vi "UHR-Fleezers Control (host) - 11.9c.vi"() -> ()   [LabVIEW 2014] (continued)
  # "Thresholds (nm)"
  # "From FX (nm)"
  # "Break?"
  # "Multiple"
  # "Bad fit"
  # "Hysteresis"
  # "Trap Trig. Fl.?"
  # "1"
  # "2"
  # "Fl. Down"
  # "Fl. Up"
  # "Bead sep"
  # "Trap Display:"
  # "APD Display:"
  # "Trap Manipulation"
  # "Data Saving"
  # "DAQ"
  # "Bead Calibration"
  # "Tether screen"
  # "Bottom Pump (#1)"
  # "Central Sample Channels"
  # "Top Pump (#3)"
  # "Rate param is ul/h\nVolume param is ul"
  # "Chemyx Pump 2"
  # "Units: \n1 = ml/m\n2 = ml/h\n3 = ul/m\n4 = ul/h"
  # "X"
  # "Y"
  # "Oscillate Set 1 freq. (debugging)"
  # "BD 1"
  # "BD 2"
  # "AOD Raster Scan"
  # "Approx. trap separations"
  # "X"
  # "Y"
  # "FPGA\nreading"
  # "DMA\ntransfer"
  # "APD Gates"
  # "APD 2"
  # "APD 1"
  # "X"
  # "2D"
  # "Y"
  # "1D"
  # "Digital Out Control"
  # "Analog Out Control (Feedback Loop)"
  # "Laser Intensity Analog Input"
  # "Total AI Rates (NOT rates/trap)"
  # "(Samples/trap x Trap Sets)"
  # "(Samples/channel x\n8 if averaging (8 channels)\n4 if no averaging)"
  # "Trap 1"
  # "Trap 2"
  # "Flour./Trap 3"
  # "External Video Window"
  # "MCL Position Debugging"
  # "Temporary Control Storage\n(these used to be somewhere else, still want to keep them)"
  # "Y"
  # "X"
  # "Trap Position Difference Limits"
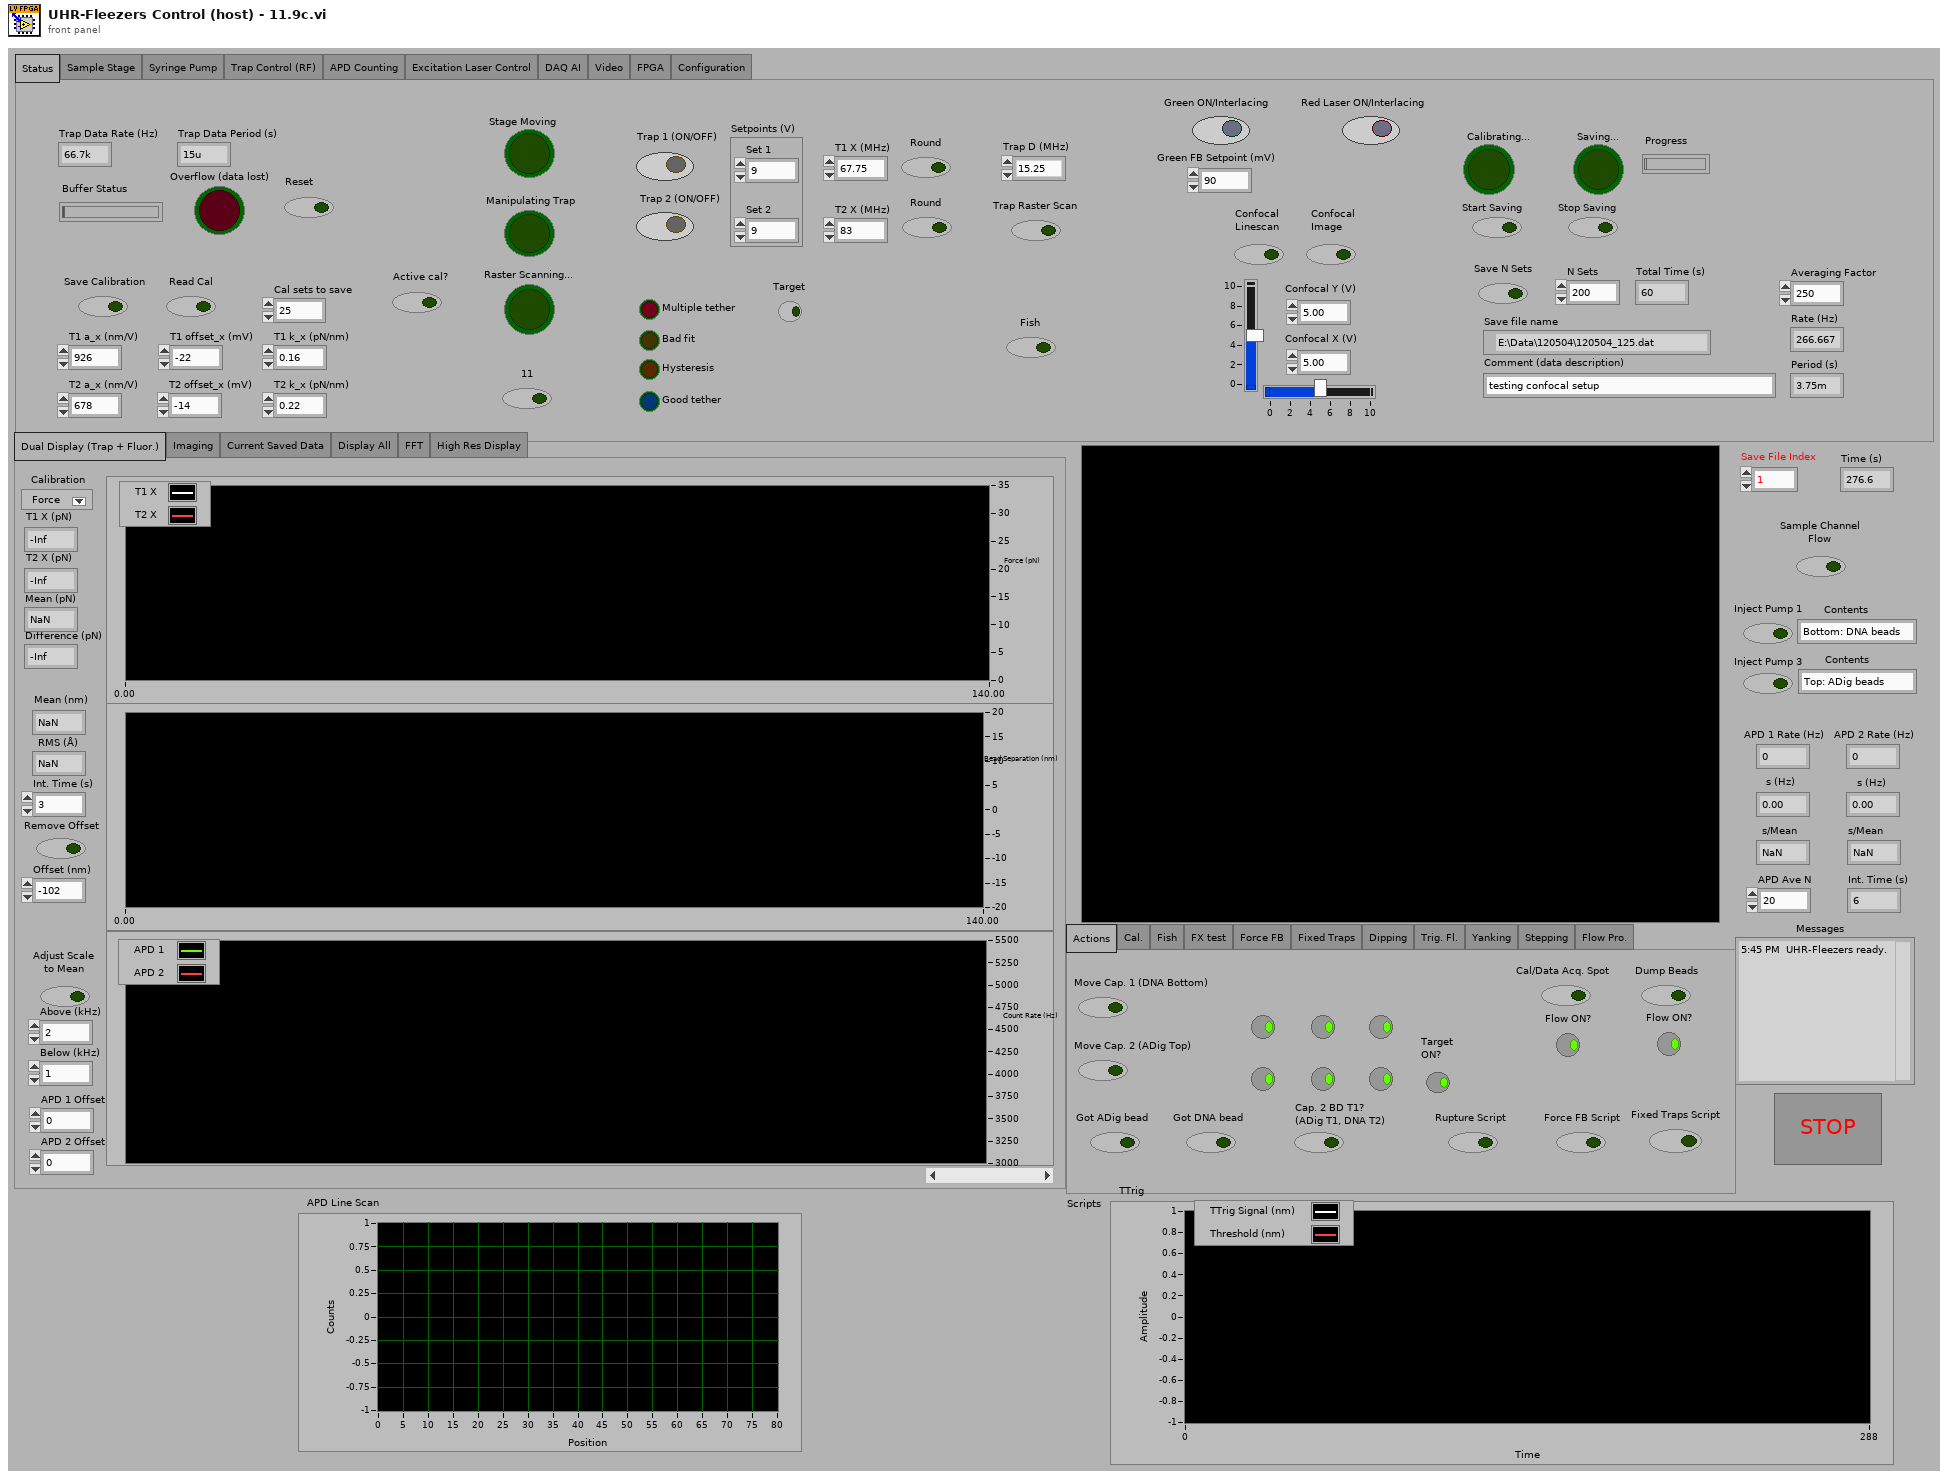
[diagram p1: front panel]
types:
  T1 = enum32{"Actions", "Cal.", "Fish", "FX test", "Force FB", "Fixed Traps", "Dipping", "Trig. Fl.", "Yanking", "Stepping", "Flow Pro."}
  T2 = typedef "IMAQ Image.ctl" = refnum<image>
  T3 = enum32{"Dual Display (Trap + Fluor.)", "Imaging", "Current Saved Data", "Display All", "FFT", "High Res Display"}
  T4 = enum32{"Status", "Sample Stage", "Syringe Pump", "Trap Control (RF)", "APD Counting", "Excitation Laser Control", "DAQ AI", "Video", "FPGA", "Configuration"}
  T5 = cluster{"Pump 1":cluster{"Diameter (mm)":dbl, "Units":dbl, "Volume":dbl, "Rate":dbl}, "Pump 2":cluster{"Diameter (mm)":dbl, "Units":dbl, "Volume":dbl, "Rate":dbl}, "Pump 3":cluster{"Diameter (mm)":dbl, "Units":dbl, "Volume":dbl, "Rate":dbl}}
  T6 = enum32{"IR Laser Interlacing (Direct RF Board Control Method)", "AOD Raster Scan", "Feedback on Trap Intensity", "Feedback on Trap Position"}
  T7 = typedef "LVPoint32TypeDef.ctl" = cluster{"Horizontal":i32, "Vertical":i32}
  T8 = cluster{"Scan Range AOD (nm) 2":dbl, "Step Size AOD (nm) 2":dbl, "Scan Speed AOD (nm/s) 2":dbl, "Number of scans (AOD) 2":u16, "Label":string}[]
  T9 = cluster{"Set 1":cluster{"proportional gain (Kc)":i16, "integral gain (Kc*Ts/Ti)":i16, "derivative gain (Kc*Td/Ts)":i16}, "Set 2":cluster{"proportional gain (Kc)":i16, "integral gain (Kc*Ts/Ti)":i16, "derivative gain (Kc*Td/Ts)":i16}}
  T10 = cluster{"Trap 1":fxp<+/-,16,1>, "Trap 2":fxp<+/-,16,1>}
  T11 = cluster{"proportional gain (Kc)":fxp<+/-,16,8>, "integral gain (Kc*Ts/Ti)":fxp<+/-,16,8>, "derivative gain (Kc*Td/Ts)":fxp<+/-,16,8>}
  T12 = cluster{"output high":fxp<+/-,64,32>, "output low":fxp<+/-,64,32>}
  T13 = cluster{"Set 1":fxp<+/-,16,1>, "Set 2":fxp<+/-,16,1>}
  T14 = enum32{"Main Controls", "Green laser (532 nm)", "Red laser (633 nm)"}
  T15 = cluster{"proportional gain (Kc)":i16, "integral gain (Kc*Ts/Ti)":i16, "derivative gain (Kc*Td/Ts)":i16}
  T16 = cluster{"Set 1":bool, "Set 2":bool, "Set 3":bool}
  T17 = typedef "LVMinMaxIncTypeDef.ctl" = cluster{"Minimum":dbl, "Maximum":dbl, "Increment":dbl}
  T18 = typedef "Image Type" = u32
  T19 = typedef "nirio_resource_hc.ctl" = tag
  T20 = typedef "openfpgaref.8.6.ctl" = refnum<k20>
  T21 = cluster{"New Image":T2, "New Image":T2, "New Image":T2, "New Image":T2}
  T22 = typedef "XDNodeRunTimeDep.lvlib/timing_clust.ctl" = cluster{"Expected End [f-1]":u64, "Actual End [f-1]":u64, "Finished Late? [f-1]":bool, "Expected End [i-1]":u64, "Actual End [i-1]":u64, "Finished Late? [i-1]":bool, "Expected Start [i]":u64, "Actual Start [i]":u64, "Expected Start [f]":u64, "Actual Start [f]":u64, "Source Name":string, "Structure Name":string, "Period":i64, "Deadline":i64, "Offset":i64, "Start":i64, "Priority":i32, "Timeout":i32, "Mode":T23, "Wakeup Reason":T24, "Error":errorcluster, "Source Type":string, "Secondary Source Type":string, "Global End Time":u64, "Global Start Time":u64, "Frame Duration":u64, "Iteration Duration":u64, "Assigned CPU":i32, "I/O Scan Engine Mode":u32}
  T23 = typedef "XDNodeRunTimeDep.lvlib/nitl_modes.ctl" = enum32{"No Change", "Process missed periods, maintain original phase", "Discard missed periods, maintain original phase", "Process missed periods, ignore original phase", "Discard missed periods, ignore original phase"}
  T24 = typedef "XDNodeRunTimeDep.lvlib/wakeup.ctl" = enum32{"Normal", "Aborted", "Asynchronous wakeup", "Timing source error", "Timed loop error", "Timeout"}
  T25 = enum16{"big-endian, network order", "native, host order", "little-endian"}
  T26 = enum16{"open", "replace", "create", "open or create", "replace or create", "replace or create with confirmation"}
  T27 = cluster{"Scan Range AOD (nm) 2":dbl, "Step Size AOD (nm) 2":dbl, "Scan Speed AOD (nm/s) 2":dbl, "Number of scans (AOD) 2":u16, "Label":string}
  T28 = cluster{"[0]":dbl, "[1]":dbl, "[2]":dbl, "[3]":dbl, "[4]":dbl, "[5]":dbl}
  T29 = cluster{"Diameter (mm)":dbl, "Units":dbl, "Volume":dbl, "Rate":dbl}
  T30 = enum16{"Actions", "Cal.", "Fish", "FX test", "Force FB", "Fixed Traps", "Dipping", "Trig. Fl.", "Yanking", "Stepping", "Flow Pro."}
  T31 = cluster{"Left":i32, "Top":i32, "Width":u32, "Height":u32}
  T32 = cluster{cluster{"Left":i32, "Top":i32, "Width":u32, "Height":u32}}[]
  T33 = enum32{"setting", "request", "request control", "info", "statistics", "system settings", "I/O sub system", "HRT control", "camera descriptions", "device specific data", "event sub system settings", "event sub system results", "image memory manager"}
  T34 = typedef "AviRefnum.ctl" = refnum<k1>
  T35 = typedef "imagedata.ctl" = cluster{"image type":i32, "image depth":i32, "image":u8[], "mask":u8[], "colors":u32[], "Rectangle":cluster{"left":i16, "top":i16, "right":i16, "bottom":i16}}
  T36 = enum32{"Normal Display", "Dual Display (APD)", "FFT", "High Res Display"}
  T37 = cluster{"Origin Pixel":cluster{"X":sgl, "Y":sgl}, "Angle Relative to Horizontal (deg)":sgl, "Axis Reference":u32}
  T38 = typedef "Simple Grid Descriptor" = cluster{"X Step":sgl, "Y Step":sgl, "Unit":T39}
  T39 = typedef "Image Unit" = enum32{"Undefined", "Angström", "Micrometer", "Millimeter", "Centimeter", "Meter", "Kilometer", "Microinch", "Inch", "Feet", "Nautical miles", "Standard miles", "Steps"}
  T40 = cluster{"averaging mode":u16, "weighting mode":u16, "number of averages":u32}
  T41 = cluster{"dB On (F)":bool, "unwrap phase (F)":bool, "convert to degree (F)":bool}
  T42 = cluster{string, string, string, string, string, string, string, string}
  T43 = cluster{string, string, string, string, string, string, string, string, string, string, string, string}
  T44 = cluster{string, string, string, string, string, string, string, string, string, string, string, string, string}
  T45 = cluster{string, string, string, string, string, string, string, string, string, string, string, string, string, string}
  T46 = cluster{"BD 1 Frequency 1 (MHz)":dbl, "BD 1 Frequency 2 (MHz)":dbl}
  T47 = cluster{"f0":dbl, "df":dbl, "magnitude":dbl[]}[][]
  T48 = cluster{"Green FB Ch 0":i16, "Green FB Ch 1":i16, "Green FB Ch 2":i16}
  T49 = cluster{"Green FB Ch 0":dbl, "Green FB Ch 1":dbl, "Green FB Ch 2":dbl}
diagram:
  w26 = 0.0 ("Total Volume\nFlowed P1 (uL)")
  w38 = u16 20 items=["1.0"=10, "1.5"=15, "2.0"=20] ("stop bits (10: 1 bit)")
  w41 = u16 20 items=["1.0"=10, "1.5"=15, "2.0"=20] ("stop bits (10: 1 bit)")
  w96 = u16 20 items=["1.0"=10, "1.5"=15, "2.0"=20] ("stop bits (10: 1 bit)")
  w103 = T18 2 items=["Grayscale (U8)", "Grayscale (I16)", "Grayscale (SGL)", "Complex (CSG)", "RGB (U32)", "HSL (U32)", "RGB (U64)", "Grayscale (U16)"] ("Image Type")
  w162 = cluster{"output high":i16, "output low":i16} {"output high"=3000, "output low"=0} ("FB output range 1")
  w233 = 10.0 ("y")
  w232 = 32767.0 ("y")
  w248 = 6.0  # clock mult.
  w249 = 49152000.0  # TCXO frequ.
  # "Safety limits on RF frequencies and amplitudes (for AOM protection)"
  # "Bottom 1 Harvard"
  # "Top 3 Harvard"
  # "Center Harvard"
  # "Bottom 1 Harvard"
  # "Top 3 Harvard"
  # "Center Harvard"
  n1 = Build Array("DIO count 1 (ticks)", "DIO count 2 (ticks)", "DIO count 3 (ticks)") -> (w149:u32[])
  n2 = local read "AO1"() -> (w227:dbl)
  n3 = local read "AO2"() -> (w226:dbl)
  n4 = local read "Scan Increment (MHz)"() -> (w244:dbl)
  n5 = local read "Continuous MCL Scanning"() -> (w214:bool)
  n6 = local read "Fast Scan Dir"() -> (w213:bool)
  n7 = local read "Number of scans (MCL)"() -> (w215:u64)
  n8 = property on="AI Count (ticks)" class="DigNum (strict)"("Val(Sgnl)"="AI Count (ticks)") -> ()  [unwired: 2 in, 2 out]
  n9 = Multiply(x=w227, y=w232) -> (x*y=w229:dbl)
  n10 = Multiply(x=w226, y=w232) -> (x*y=w231:dbl)
  n11 = Divide(x=w229, y=w233) -> (x/y=w228:dbl)
  n12 = Divide(x=w231, y=w233) -> (x/y=w230:dbl)
  n13 = To Word Integer(number=w228) -> (16bit integer=w225:i16)
  n14 = To Word Integer(number=w230) -> (16bit integer=w224:i16)
  n15 = Not(x=w213) -> (.not. x?=w208:bool)
  n16 = local read "Cycles/step (MCL)"() -> (w216:u64)
  n17 = Multiply(x=w244, y=1000.0) -> (x*y=w251:dbl)
  n18 = local read "Scan steps (MCL)"() -> (w217:u64)
  n19 = local write "Trap Pos FIFO Timeout"(u16 0 ("Trap Pos FIFO Timeout")) -> ()
  n20 = local read "Desired Scan Incr (V)"() -> (w219:dbl)
  n21 = Scale By Power Of 2(n=48, x=w251) -> (x*2^n=w252:dbl)
  n22 = Multiply(x=w249, y=w248) -> (x*y=w247:dbl)
  n23 = Divide(x=w252, y=w247) -> (x/y=w246:dbl)
  n24 = local read "Setpoints (V)"() -> (w263:cluster{"Set 1":dbl, "Set 2":dbl})
  n25 = To Quad Integer(1:w246) -> (0:w243:i64)
  n26 = Divide(x=40000000.0, y="AI Count (ticks)") -> (x/y=w204:dbl)
  n27 = Multiply(x=w219, y=32767.0) -> (x*y=w221:dbl)
  n28 = local read "Number Interlace Sets"() -> (w142:u8)
  n29 = Split 1D Array(array=w149, index=w142) -> (first subarray=w151:u32[])  [unwired: 1 out]
  n30 = Add Array Elements(numeric array=w151) -> (sum=w150:u32)
  n31 = local read "# Samples/channel"() -> (w236:u32)
  n32 = local read "Number of F/B Scans (AOD)"() -> (w237:u16)
  n33 = local read "Not-Interlacing Set"() -> (w141:enum32{"Set 1", "Set 2", "Set 3"})
  n34 = To Unsigned Byte Integer(number=w141) -> (unsigned 8bit integer=w147:u8)
  n35 = Index Array(array=w149, index=w147) -> (element=w148:u32)
  n36 = local read "Feedback On/Off"() -> (w266:cluster{"Set 1":bool, "Set 2":bool})
  n37 = local read "PID Gains"() -> (w258:T9)
  n38 = local read "Scan steps (AOD)"() -> (w242:u64)
  n39 = local read "All FB On/Off"() -> (w267:bool)
  n40 = local read "Cycles/step (AOD)"() -> (w241:u64)
  n41 = local write "AI rate (Hz)"(w204) -> ()
  n42 = Divide(x=w221, y=10.0) -> (x/y=w220:dbl)
  n43 = Multiply(x=w242, y=w241) -> (x*y=w240:u64)
  n44 = Multiply(x=3276.7, y=w263) -> (x*y=w262:cluster{"Set 1":dbl, "Set 2":dbl})
  n45 = To Word Integer(number=w220) -> (16bit integer=w218:i16)
  n46 = xnode "Open FPGA VI Reference"("resource name"=T19 "RIO1") -> ("FPGA VI Reference Out"=w24:T20, "error out"=w22:errorcluster)  [unwired: 1 in]
  n47 = Multiply(x=w240, y=u64 2) -> (x*y=w238:u64)
  n48 = local read "Sets to FIFO (Traps)"() -> (w270:T16)
  n49 = Divide(x=w204, y="FPGA Ave.") -> (x/y=w205:dbl)
  n50 = To Word Integer(number=w262) -> (16bit integer=w261:cluster{"Set 1":i16, "Set 2":i16})
  n51 = Unbundle By Name(w258) -> ("Set 1"=w257:T15, "Set 2"=w256:T15)
  n52 = Multiply(x=w238, y=w237) -> (x*y=w235:u64)
  n53 = local write "Ave. Rate (Hz)"(w205) -> ()
  n54 = Divide(x=w235, y=w236) -> (x/y=w234:dbl)
  n55 = Unbundle By Name(w261) -> ("Set 1"=w260:i16, "Set 2"=w259:i16)
  n56 = local read "2D or 1D Scan"() -> (w163:bool)
  n57 = local write "Data points/scans"(w235) -> ()
  n58 = local read "Scan BD"() -> (w253:bool)
  n59 = And(x=w266, y=w267) -> (x .and. y?=w265:cluster{"Set 1":bool, "Set 2":bool})
  n60 = local write "Data points/scan (f/b)"(w238) -> ()
  n61 = Reciprocal(x=w205) -> (1/x=w206:dbl)
  n62 = local read "N Acq Sets (Traps + Fl.)"() -> (w197:i16)
  n63 = local write "N sets should be saved"(w234) -> ()
  n64 = xnode "Invoke Method"("FPGA VI Reference In"=w24, "error in"=w22) -> ("FPGA VI Reference Out"=w161:T20, "error out"=w171:errorcluster)
  n65 = Unbundle By Name(w265) -> ("Set 1"=w269:bool, "Set 2"=w268:bool)
  n66 = local read "Interlace"() -> (w143:bool)
  n67 = Select(t=w150, s=w143, f=w148) -> (s? t:f=w140:u32)
  n68 = local write "Update Count (MCL)"(w140) -> ()
  n69 = local write "Total Counts (ticks)"(w140) -> ()
  n70 = local write "Ave. Period (s)"(w206) -> ()
  n71 = property on="2D or 1D Scan" class="Bool (strict)"("Val(Sgnl)"=w163) -> ()  [unwired: 2 in, 2 out]
  n72 = local read "APD Gate OFF Count"() -> (w65:u16)
  n73 = local read "Interlace OFF count"() -> (w68:u16)
  n74 = local read "Interlace ON count"() -> (w3:u16)
  n75 = local read "APD Gate ON Count"() -> (w61:u16)
  n76 = xnode "Read/Write Control"("FPGA VI Reference In"=w160, "error in"=w171, "ai count"="AI Count (ticks)", "Interlace ON/OFF"=w143, "Number Interlace Cycles"=w142, "AI1 Sets to FIFO"=w270, "FB On/Off Set 1"=w269, "FB On/Off Set 2"=w268, "Interlace Off Parameters"=w141, "FB Setpoint Set 1"=w260, "FB Setpoint Set 2"=w259, "FB Gains Set 1"=w257, "FB Gains Set 2"=w256, "FB output range 1"=w162, "FB output range 2"=w162, "Cycles per step"=w241, "Scan BD"=w253, "Number of scans"=w237, "Scan steps"=w242, "Scan freq.  increment"=w243, "AO1"=w225, "AO2"=w224, "Scan freq.  increment (MCL)"=w218, "Scan steps (MCL)"=w217, "Cycles per step (MCL)"=w216, "Number of scans (MCL)"=w215, "MCL count"=w140, "Cont. Scan (MCL)"=w214, "MCL Scan Axis"=w208, "1D or 2D Scan?"=w163, "N of AI1 Int Acq Sets"=w197, "Freq or Amp switch first"="Freq or Amp switch first", "Freq switch delay"="Freq switch delay", "Amp switch delay"="Amp switch delay", "Swap F1 and F2"="Swap F1 and F2", "APD to FIFO"=FALSE, "DIO count 1 (ticks)"="DIO count 1 (ticks)", "DIO count 2 (ticks)"="DIO count 2 (ticks)", "DIO count 3 (ticks)"="DIO count 3 (ticks)") -> ("FPGA VI Reference Out"=w72:T20, "error out"=w70:errorcluster)  [unwired: 1 in]
  n77 = local read "Duty frequency (ON 1/N cycles)"() -> (w67:u16)
  n78 = local read "APD Integration Time (s)"() -> (w53:dbl)
  n79 = local read "DMA Update Period (s)"() -> (w52:dbl)
  n80 = local read "Red Laser ON/Interlacing"() -> (w6:bool)
  n81 = Add(x=w61, y=w65) -> (x+y=w63:u16)
  n82 = local read "Laser interlacing mode (all lasers)"() -> (w5:enum32{"Laser ON", "Laser OFF", "Interlace"})
  n83 = Add(x=w3, y=w68) -> (x+y=w66:u16)
  n84 = local read "Green ON/Interlacing"() -> (w139:bool)
  n85 = Multiply(x=w63, y=w67) -> (x*y=w64:u16)
  n86 = Multiply(x=w67, y=w66) -> (x*y=w60:u16)
  n87 = Reciprocal(x=w53) -> (1/x=w50:dbl)
  n88 = Multiply(x=w53, y=40000000.0) -> (x*y=w49:dbl)
  n89 = Divide(x=w52, y=w53) -> (x/y=w55:dbl)
  n90 = Multiply(x="Green intensity % (FB OFF)", y=655.35) -> (x*y=w129:dbl)
  n91 = local read "Invert laser interlacing"() -> (w1:bool)
  n92 = case shown="False" w6 {
    tunnel: w5 -> [_ w295]
    tunnel: [enum32{"Laser ON", "Laser OFF", "Interlace"}."Laser OFF" ("Laser interlacing mode (all lasers)") w295] -> w4
    frame False {
    }
    frame True {
    }
  }
  n93 = local read "Invert APD Gate"() -> (w59:bool)
  n94 = Multiply(x="Green FB Setpoint (mV)", y=3.2767) -> (x*y=w126:dbl)
  n95 = local read "APD Gate"() -> (w58:enum32{"ON", "OFF", "Interlace"})
  n96 = Subtract(x=w64, y=w61) -> (x-y=w62:u16)
  n97 = local write "Green FB Count"(w60) -> ()
  n98 = local write "APD Acq Rate (Hz)"(w50) -> ()
  n99 = To Unsigned Long Integer(number=w49) -> (unsigned 32bit integer=w47:u32)
  n100 = Multiply(x=2.0, y=w55) -> (x*y=w54:dbl)
  n101 = To Unsigned Word Integer(number=w129) -> (unsigned 16bit integer=w127:u16)
  n102 = Subtract(x=w60, y=w3) -> (x-y=w2:u16)
  n103 = local write "APD Samples/FIFO Acq."(w55) -> ()
  n104 = To Word Integer(number=w126) -> (16bit integer=w124:i16)
  n105 = local write "APD Elements/DMA read"(w54) -> ()
  n106 = case shown="False" w139 {
    tunnel: w5 -> [_ w297]
    tunnel: [enum32{"Laser ON", "Laser OFF", "Interlace"}."Laser OFF" ("Green laser mode") w297] -> w7
    frame False {
    }
    frame True {
    }
  }
  n107 = local write "APD Int. Count"(w47) -> ()
  n108 = Multiply(x="Red intensity % (FB OFF)", y=655.35) -> (x*y=w11:dbl)
  n109 = local read "Trap Pos. AI1 X Pre-scale"() -> (w82:u16)
  n110 = local read "Trap Pos FB Monitor\nT1 or T2"() -> (w89:bool)
  n111 = To Unsigned Word Integer(number=w11) -> (unsigned 16bit integer=w10:u16)
  n112 = local read "Trap Pos FB Int Count"() -> (w76:u16)
  n113 = local read "APD 1 AO Mult."() -> (w57:i16)
  n114 = local read "Trap Pos FB Negate Action"() -> (w88:bool)
  n115 = local read "APD 2 AO Mult."() -> (w56:i16)
  n116 = local read "Trap Pos. FB Offset Factor"() -> (w87:i64)
  n117 = local read "Trap Pos. FB Mult Factor"() -> (w86:i64)
  n118 = local read "Differential FB?"() -> (w44:bool)
  n119 = local read "Neg. TTrig FPGA"() -> (w46:bool)
  n120 = local read "Trap Pos. FB Gains"() -> (w84:T11)
  n121 = local read "Trap Pos. FB Range"() -> (w85:T12)
  n122 = xnode "Read/Write Control"("FPGA VI Reference In"=w72, "error in"=w70, "Invert APD Gate"=w59, "APD Gate ON Count"=w61, "APD Gate OFF Count"=w62, "APD Acq Rate Count"=w47, "APD Gate Operating Mode"=w58, "APD 1 AO scale factor"=w57, "APD 2 AO scale factor"=w56, "Green interlace ON count"=w3, "Green interlace OFF count"=w2, "Green interlace ON count 2"=w3, "Green interlace OFF count 2"=w2, "Green FB Count"=w60, "RI ON count"=w3, "RI OFF count"=w2) -> ("FPGA VI Reference Out"=w71:T20, "error out"=w69:errorcluster)
  n123 = xnode "Read/Write Control"("FPGA VI Reference In"=w71, "error in"=w69, "Invert GI 2"=w1, "Operating Mode 2"=w7, "Green FB Gains"="Green FB Gains", "Green FB Setpoint"=w124, "Green FB On/Off"="Green FB On/Off", "Current Out"=w127, "Green int current ON count adj"="Green int current ON count adj", "Operating Mode"=w7, "Invert GI"=w1, "Trap Pos FB Monitor T1 or T2"=w89, "Trap Pos FB Negate Action"=w88, "Trap Pos. FB Offset Factor"=w87, "Trap Pos. FB Mult Factor"=w86, "Trap Pos. FB Range"=w85, "Trap Pos. FB Gains"=w84, "Force feedback"=FALSE, "AI1 X Scale"=w82, "Trap Pos to FIFO"=TRUE, "Trap Pos FB Int Count"=w76, "TTrig Negate Pos"=w46, "FB Trig Integrate"="FB Trig Integrate", "Diff FB Measurement?"=w44, "Negate Diff?"="Negate Diff?", "RI Current Out"=w10, "Red operating mode"=w4, "RI operating mode 2"=w4, "Invert RI"=w1, "Invert RI 2"=w1) -> ("FPGA VI Reference Out"=w137:T20, "error out"=w138:errorcluster)
  n124 = xnode "Invoke Method"("FPGA VI Reference In"=w137, "error in"=w138, "Requested Depth"="Trap AI FIFO Depth") -> ("FPGA VI Reference Out"=w92:T20, "error out"=w91:errorcluster)  [unwired: 1 out]
  n125 = xnode "Invoke Method"("FPGA VI Reference In"=w92, "error in"=w91, "Requested Depth"="Trap Position FIFO Depth") -> ("FPGA VI Reference Out"=w78:T20, "error out"=w77:errorcluster)  [unwired: 1 out]
  n126 = flat-sequence {
    tunnel: w161 -> [w302]
    tunnel: [w302] -> w160
    tunnel: [w301] -> w159
    tunnel: [w300] -> w158
    tunnel: [w298] -> w156
    tunnel: [w299] -> w157
    frame #0 {
      w299 = T17 {"Minimum"=0.0, "Maximum"=40.0, "Increment"=1.0} ("Min Max Inc")
      w298 = T17 {"Minimum"=0.0, "Maximum"=50.0, "Increment"=1.0} ("Data Entry Limits")
      w301 = T17 {"Minimum"=60.0, "Maximum"=90.0, "Increment"=1.0} ("Min Max Inc")
      w300 = T17 {"Minimum"=0.0, "Maximum"=50.0, "Increment"=1.0} ("Data Entry Limits")
      n127 = property on="BD 2 Frequency 1 (MHz)" class="DigNum (strict)"("Data Range"=w299) -> ()  [unwired: 2 in, 2 out]
      n128 = property on="BD 2 Frequency 3 (MHz)" class="DigNum (strict)"("Data Range"=w299) -> ()  [unwired: 2 in, 2 out]
      n129 = property on="BD 2 Frequency 2 (MHz)" class="DigNum (strict)"("Data Range"=w299) -> ()  [unwired: 2 in, 2 out]
      n130 = property on="BD 1 Frequency 1 (MHz)" class="DigNum (strict)"("Data Range"=w301) -> ()  [unwired: 2 in, 2 out]
      n131 = property on="BD 1 Frequency 2 (MHz)" class="DigNum (strict)"("Data Range"=w301) -> ()  [unwired: 2 in, 2 out]
      n132 = property on="BD 1 Frequency 3 (MHz)" class="DigNum (strict)"("Data Range"=w301) -> ()  [unwired: 2 in, 2 out]
      n133 = property on="BD 2 Amplitude 1 (%)" class="DigNum (strict)"("Data Range"=w298) -> ()  [unwired: 2 in, 2 out]
      n134 = property on="BD 2 Amplitude 2 (%)" class="DigNum (strict)"("Data Range"=w298) -> ()  [unwired: 2 in, 2 out]
      n135 = property on="BD 2 Amplitude 3 (%)" class="DigNum (strict)"("Data Range"=w298) -> ()  [unwired: 2 in, 2 out]
      n136 = property on="BD 1 Amplitude 3 (%)" class="DigNum (strict)"("Data Range"=w300) -> ()  [unwired: 2 in, 2 out]
      n137 = property on="BD 1 Amplitude 2 (%)" class="DigNum (strict)"("Data Range"=w300) -> ()  [unwired: 2 in, 2 out]
      n138 = property on="BD 1 Amplitude 1 (%)" class="DigNum (strict)"("Data Range"=w300) -> ()  [unwired: 2 in, 2 out]
      "X RF Frequency Limits (MHz)" <- w301
      "X RF Amplitude Limits (%)" <- w300
      "Y RF Amplitude Limits (%)" <- w298
      "Y RF Frequency Limits (MHz)" <- w299
    }
  }
  n139 = xnode "Invoke Method"("FPGA VI Reference In"=w78, "error in"=w77) -> ("FPGA VI Reference Out"=w170:T20, "error out"=w169:errorcluster)  [unwired: 1 in]
  n140 = flat-sequence "Initial FPGA Loop Relative Phase Adjustment" {
    tunnel: "Initial Phase Adjustment (APD 2 Gate)" -> [w305]
    tunnel: "Initial Phase Adjust (GI) 2" -> [w306]
    tunnel: "Initial Phase Adj. (MCL)" -> [w304]
    tunnel: w169 -> [w307]
    tunnel: w170 -> [w308]
    tunnel: "Initial Phase Adjust (GI)" -> [w309]
    tunnel: "Initial Phase Adjustment (AI1)" -> [w310]
    tunnel: [w310] -> w21
    tunnel: [w309] -> w20
    tunnel: [w308] -> w19
    tunnel: [w307] -> w18
    tunnel: [w304] -> w17
    tunnel: [w306] -> w16
    tunnel: [w305] -> w15
    tunnel: [w323] -> w179
    tunnel: [w317] -> w175
    tunnel: "Initial Phase Adjustment (APD Acq)" -> [w316]
    tunnel: "Initial Phase Adjustment (APD 1 Gate)" -> [w315]
    tunnel: "Initial Phase Adjust (Green FB)" -> [w314]
    tunnel: w21 -> [w322]
    tunnel: w20 -> [w321]
    tunnel: w19 -> [w320]
    tunnel: w18 -> [w319]
    tunnel: w17 -> [w318]
    tunnel: w16 -> [w313]
    tunnel: w15 -> [w312]
    tunnel: "Initial Phase Adjustment (RI)" -> [w311]
    tunnel: w179 -> [w325]
    tunnel: [w326] -> w176
    tunnel: w175 -> [w326]
    tunnel: [w325] -> w174
    tunnel: w176 -> [w329]
    tunnel: w174 -> [w328]
    tunnel: [w331] -> w173
    tunnel: [w330] -> w172
    tunnel: [w333] -> w177
    tunnel: [w334] -> w178
    tunnel: w173 -> [w334]
    tunnel: w172 -> [w333]
    frame #0 {
      n141 = Wait (ms)(milliseconds to wait=u32 100) -> ()  [unwired: 1 out]
    }
    frame #1 {
      n142 = xnode "Read/Write Control"("FPGA VI Reference In"=w320, "error in"=w319, "Phase count adjustment"=w322, "Phase count adjustment (GI)"=w321, "Phase count adjustment (MCL)"=w318, "Phase Count Adjustment (APD Acq)"=w316, "Phase count adjustment (APD 1 Gate)"=w315, "Phase count adjustment (APD 2 Gate)"=w312, "Phase count adjustment (Green FB)"=w314, "Phase count adjustment (GI) 2"=w313, "Phase count adjustment (RI)"=w311) -> ("FPGA VI Reference Out"=w317:T20, "error out"=w323:errorcluster)
    }
    frame #2 {
      n143 = Wait (ms)(milliseconds to wait=u32 100) -> ()  [unwired: 1 out]
    }
    frame #3 {
      w327 = TRUE
      n144 = xnode "Read/Write Control"("FPGA VI Reference In"=w329, "error in"=w328, "+ phase"=w327, "+ phase (GI)"=w327, "+ phase (MCL)"=w327, "+ phase (APD Acq)"=w327, "+ phase (APD 1 Gate)"=w327, "+ phase (APD 2 Gate)"=w327, "+ phase (Green FB)"=w327, "+ phase (GI) 2"=w327, "+ phase (RI)"=w327) -> ("FPGA VI Reference Out"=w330:T20, "error out"=w331:errorcluster)
    }
    frame #4 {
      n145 = Wait (ms)(milliseconds to wait=u32 100) -> ()  [unwired: 1 out]
    }
  }
  n146 = local read "Phase adj. (Green FB)"() -> (w152:i16)
  n147 = local read "Phase adj. (GI) 2"() -> (w130:i16)
  n148 = local read "Phase adj. (RI)"() -> (w8:i16)
  n149 = local read "Phase adjust (MCL)"() -> (w209:i16)
  n150 = local read "Phase adj. (AI1)"() -> (w211:i16)
  n151 = local read "Phase adj. (GI)"() -> (w210:i16)
  n152 = xnode "Read/Write Control"("FPGA VI Reference In"=w177, "error in"=w178, "Phase count adjustment"=w211, "Phase count adjustment (GI)"=w210, "Phase count adjustment (MCL)"=w209, "Phase Count Adjustment (APD Acq)"="Phase Adj. (APD Acq)", "Phase count adjustment (APD 1 Gate)"="Phase Adj. (APD 1 Gate)", "Phase count adjustment (APD 2 Gate)"="Phase Adj. (APD 2 Gate)", "Phase count adjustment (Green FB)"=w152, "Phase count adjustment (GI) 2"=w130, "Phase count adjustment (RI)"=w8) -> ("FPGA VI Reference Out"=w23:T20, "error out"=w186:errorcluster)
  n153 = call "Initialize RF boards - interlace 3.vi"("error in"=w186, "FPGA VI Reference In"=w23) -> ("error out"=w184:errorcluster, "FPGA VI Reference Out"=w185:T20)
  n154 = call "set RF board frequency - interlace.vi"("Board 2 Frequency Limits"=w157, "Board 1 Frequency Limits"=w159, "error in"=w184, "FPGA VI Reference In"=w185, "Board 2 Frequency 3 (MHz)"="BD 2 Frequency 3 (MHz)", "Board 1 Frequency 3 (MHz)"="BD 1 Frequency 3 (MHz)", "Board 2 Frequency 2 (MHz)"="BD 2 Frequency 2 (MHz)", "Board 2 Frequency 1 (MHz)"="BD 2 Frequency 1 (MHz)", "Board 1 Frequency 2 (MHz)"="BD 1 Frequency 2 (MHz)", "Board 1 Frequency 1  (MHz)"="BD 1 Frequency 1 (MHz)") -> ("error out"=w285:errorcluster, "FPGA VI Reference Out"=w286:T20)
  n155 = call "set RF board amplitude - interlace.vi"("Board 2 Amplitude Limits"=w156, "Board 1 Amplitude Limits"=w158, "error in"=w285, "FPGA VI Reference In"=w286, "Board 2 Amplitude 3 (%)"="BD 2 Amplitude 3 (%)", "Board 1 Amplitude 3 (%)"="BD 1 Amplitude 3 (%)", "Board 2 Amplitude 2 (%)"="BD 2 Amplitude 2 (%)", "Board 2 Amplitude 1 (%)"="BD 2 Amplitude 1 (%)", "Board 1 Amplitude 2 (%)"="BD 1 Amplitude 2 (%)", "Board 1 Amplitude 1 (%)"="BD 1 Amplitude 1 (%)") -> ("error out"=w273:errorcluster, "FPGA VI Reference Out"=w274:T20)
  n156 = flat-sequence {
    tunnel: w274 -> [w344]
    tunnel: w273 -> [w343]
    tunnel: [w342] -> w278
    tunnel: [w341] -> w277
    tunnel: [w348] -> w276
    tunnel: w278 -> [w348]
    tunnel: [w347] -> w275
    tunnel: w277 -> [w347]
    tunnel: w276 -> [w357]
    tunnel: w275 -> [w356]
    tunnel: [w355] -> w32
    tunnel: [w354] -> w79
    frame #0 {
      w335 = FALSE ("Retract Pump 3")
      n157 = local read "Trap 1 (ON/OFF)"() -> (w336:bool)
      n158 = xnode "Read/Write Control"("FPGA VI Reference In"=w344, "error in"=w343, "Direct RF Box  Communication"=FALSE) -> ("FPGA VI Reference Out"=w342:T20, "error out"=w341:errorcluster)
      n159 = local write "Saving..."(FALSE ("Saving Data")) -> ()
      n160 = local write "Stop All"(FALSE ("Stop All")) -> ()
      n161 = local write "Retract Pump 1"(w335) -> ()
      n162 = local write "Retract Pump 3"(w335) -> ()
      n163 = local write "Index"(1.0 ("Index")) -> ()
      n164 = property on="Trap 1 ON" class="Bool (strict)"("Value"=w336) -> ()  [unwired: 2 in, 2 out]
      "Manipulating Trap" <- FALSE ("Manipulating Trap")
    }
    frame #1 {
      n165 = local read "Trap 2 (ON/OFF)"() -> (w346:bool)
      n166 = Wait (ms)(milliseconds to wait=u32 10) -> ()  [unwired: 1 out]
      n167 = property on="Trap 2 ON" class="Bool (strict)"("Val(Sgnl)"=w346) -> ()  [unwired: 2 in, 2 out]
    }
    frame #2 {
      n168 = local read "Scan Range (nm)"() -> (w350:dbl)
      n169 = xnode "Read/Write Control"("FPGA VI Reference In"=w357, "error in"=w356, "FPGA Controls  RF Box"=TRUE ("Direct RF Box  Communication")) -> ("FPGA VI Reference Out"=w355:T20, "error out"=w354:errorcluster)
      n170 = call "Update messages.vi"("Message to add"="UHR-Fleezers ready.", "Old message string"="") -> ("New message string"=w353:string)
      n171 = local write "Messages"(w353) -> ()
      n172 = property on="Scan Range (nm)" class="DigNum (strict)"("Val(Sgnl)"=w350) -> ()  [unwired: 2 in, 2 out]
    }
  }
  n173 = Subtract(x="BD 1 Frequency 1 (MHz)", y="BD 1 Frequency 2 (MHz)") -> (x-y=w196:dbl)
  n174 = Subtract(x="BD 2 Frequency 1 (MHz)", y="BD 2 Frequency 2 (MHz)") -> (x-y=w195:dbl)
  n175 = Square(x=w195) -> (x^2=w193:dbl)
  n176 = Square(x=w196) -> (x^2=w194:dbl)
  n177 = Add(x=w194, y=w193) -> (x+y=w192:dbl)
  n178 = Square Root(x=w192) -> (sqrt(x)=w191:dbl)
  n179 = local write "Trap D (MHz)"(w191) -> ()
  n180 = call "IMAQ Create"("Image Name"="APD 1 Image", "Image Type"=w103) -> ("New Image"=w102:T2)  [unwired: 3 in, 1 out]
  n181 = call "IMAQ Create"("Image Name"="APD 2 Image", "Image Type"=w103) -> ("New Image"=w101:T2)  [unwired: 3 in, 1 out]
  n182 = call "IMAQ Create"("Image Name"="Det. X Image", "Image Type"=w103) -> ("New Image"=w100:T2)  [unwired: 3 in, 1 out]
  n183 = call "IMAQ Create"("Image Name"="Det. Y Image", "Image Type"=w103) -> ("New Image"=w99:T2)  [unwired: 3 in, 1 out]
  n184 = Bundle("New Image"=w102, "New Image"=w101, "New Image"=w100, "New Image"=w99) -> (w98:T21)  [unwired: 1 in]
  n185 = call-poly "VISA Configure Serial Port"("VISA resource name"="Bottom  1 Harvard Syringe Pump Serial Port", "baud rate (9600)"=u32 115200, "stop bits (10: 1 bit)"=w38) -> ("VISA resource name out"=w34:refnum<visa-resource-name>, "error out"=w33:errorcluster)  [unwired: 4 in, 7 out]
  n186 = call-poly "VISA Configure Serial Port"("VISA resource name"="Top 3 Harvard Syringe Pump Serial Port", "baud rate (9600)"=u32 115200, "stop bits (10: 1 bit)"=w41) -> ("VISA resource name out"=w36:refnum<visa-resource-name>, "error out"=w35:errorcluster)  [unwired: 4 in, 7 out]
  n187 = call-poly "VISA Configure Serial Port"("VISA resource name"="Sample Chamber Stage Serial Port") -> ("VISA resource name out"=w112:refnum<visa-resource-name>, "error out"=w113:errorcluster)  [unwired: 5 in, 8 out]
  "Stage Control Serial Error" <- w113
  n188 = call-poly "VISA Configure Serial Port"("VISA resource name"="Center Harvard Syringe Pump Serial Port", "baud rate (9600)"=u32 115200, "stop bits (10: 1 bit)"=w96) -> ("VISA resource name out"=w93:refnum<visa-resource-name>, "error out"=w94:errorcluster)  [unwired: 4 in, 7 out]
  n189 = disable-structure shown="Disabled" {
    disable-tunnel: [w360 _] -> w255
    disable-tunnel: w32 -> [w359 _]
    frame Disabled {
      n190 = node-c288() -> (w362:T22)  [unwired: 4 out]
      n191 = timed-loop "Rough control of MCL mirror stage (debugging)" {
        tunnel: w359 -> [w365]
        tunnel: [w364] -> w360
        timing: w362 -> [_]
        timing-out: [_] -> w361
        stop <- w364 stop-if-true
        n192 = node-c288() -> ()  [unwired: 2 out]
        n193 = case shown="1" "MCL Mode" {
          tunnel: w365 -> [_ w368 w415]
          frame 0, Default {
          }
          frame 1 {
            n194 = node-c288() -> (w370:T22)  [unwired: 4 out]
            n195 = timed-loop "Oscillate MCL mirror" {
              timing: w370 -> [_]
              timing-out: [_] -> w369
              tunnel: w368 -> [w409]
              i -> [w408]
              stop <- w371 stop-if-true
              n196 = node-c288() -> (w407:i64)  [unwired: 1 out]
              n197 = Multiply(x="AO1", y=32767.0) -> (x*y=w403:dbl)
              n198 = Multiply(x="AO2", y=32767.0) -> (x*y=w398:dbl)
              n199 = Divide(x=w403, y=10.0) -> (x/y=w404:dbl)
              n200 = Divide(x=w398, y=10.0) -> (x/y=w399:dbl)
              n201 = To Word Integer(number=w404) -> (16bit integer=w396:i16)
              n202 = To Word Integer(number=w399) -> (16bit integer=w395:i16)
              n203 = Divide(x=w407, y=i64 1000) -> (x/y=w378:dbl)
              n204 = Multiply(x=w378, y=w408) -> (x*y=w389:dbl)
              n205 = Multiply(x="Osc. freq. (Hz) 2", y=6.283185307179586) -> (x*y=w390:dbl)
              n206 = Multiply(x=w390, y=w389) -> (x*y=w388:dbl)
              n207 = Sine(x=w388) -> (sin(x)=w387:dbl)
              n208 = Multiply(x=w387, y="Osc. amp. (V)") -> (x*y=w385:dbl)
              n209 = Add(x=w385, y="Osc. center (V)") -> (x+y=w383:dbl)
              n210 = Divide(x=w383, y=10.0) -> (x/y=w381:dbl)
              n211 = Multiply(x=w381, y=32767.0) -> (x*y=w376:dbl)
              n212 = Select(t=w376, s="Scan axis", f=w396) -> (s? t:f=w394:dbl)
              n213 = Select(t=w395, s="Scan axis", f=w376) -> (s? t:f=w393:dbl)
              n214 = local read "MCL Mode"() -> (w375:u16)
              n215 = Not Equal?(x=w375, y=u16 1) -> (x != y?=w372:bool)
              n216 = local read "Stop All"() -> (w373:bool)
              n217 = xnode "Read/Write Control"("FPGA VI Reference In"=w409, "AO1"=w394, "AO2"=w393) -> ()  [unwired: 1 in, 2 out]
              n218 = Compound Arithmetic op=OR(w373, w372) -> (w371:bool)
              n219 = node-c288() -> ()  [unwired: 2 out]
            }
            n220 = node-c288(w369) -> ()  [unwired: 1 out]
          }
          frame 2 {
            n221 = case shown="True" "Start Scan" {
              tunnel: w415 -> [_ w427]
              frame False {
              }
              frame True {
                n222 = Subtract(x="End (V)", y="Begin (V)") -> (x-y=w423:dbl)
                n223 = Decrement(x="N Points") -> (x-1=w422:dbl)
                n224 = Divide(x=w423, y=w422) -> (x/y=w420:dbl)
                n225 = for {
                  N: "N Points" -> [_]
                  tunnel: "Begin (V)" -> [w440]
                  tunnel: w427 -> [w432]
                  tunnel: [w431] -> w426 mode=indexing
                  tunnel: w420 -> [w430]
                  tunnel: [w428] -> w419 mode=indexing
                  i -> [w439]
                  n226 = Multiply(x=w430, y=w439) -> (x*y=w438:dbl)
                  n227 = Add(x=w440, y=w438) -> (x+y=w435:dbl)
                  n228 = local read "Scan axis"() -> (w429:bool)
                  n229 = local read "AO1"() -> (w437:dbl)
                  n230 = local read "AO2"() -> (w436:dbl)
                  n231 = Select(t=w435, s=w429, f=w437) -> (s? t:f=w434:dbl)
                  n232 = Select(t=w436, s=w429, f=w435) -> (s? t:f=w433:dbl)
                  n233 = flat-sequence {
                    tunnel: w434 -> [w444]
                    tunnel: w433 -> [w443]
                    tunnel: w432 -> [w441]
                    tunnel: [w454] -> w431
                    tunnel: [w453] -> w428
                    frame #0 {
                      w447 = 10.0 ("y")
                      w442 = 32767.0 ("y")
                      n234 = Multiply(x=w444, y=w442) -> (x*y=w450:dbl)
                      n235 = Multiply(x=w443, y=w442) -> (x*y=w448:dbl)
                      n236 = Divide(x=w450, y=w447) -> (x/y=w451:dbl)
                      n237 = Divide(x=w448, y=w447) -> (x/y=w449:dbl)
                      n238 = To Word Integer(number=w451) -> (16bit integer=w445:i16)
                      n239 = To Word Integer(number=w449) -> (16bit integer=w446:i16)
                      n240 = xnode "Read/Write Control"("FPGA VI Reference In"=w441, "AO1"=w445, "AO2"=w446) -> ()  [unwired: 1 in, 2 out]
                    }
                    frame #1 {
                      n241 = Wait (ms)(milliseconds to wait="DAQ Delay (ms)") -> ()  [unwired: 1 out]
                    }
                    frame #2 {
                      n242 = local read "Slow mean"() -> (w454:dbl)
                      n243 = local read "Sigma"() -> (w453:dbl)
                    }
                  }
                }
                n244 = Bundle("Begin (V)"="Begin (V)", w420, w426) -> (→"MCL Scan":cluster{"Begin (V)":dbl, dbl, dbl[]})  [unwired: 1 out]
                n245 = Bundle("Begin (V)"="Begin (V)", w420, w419) -> (→"MCL Scan 2":cluster{"Begin (V)":dbl, dbl, dbl[]})  [unwired: 1 out]
              }
            }
          }
        }
        n246 = local read "Stop All"() -> (w364:bool)
        n247 = node-c288() -> ()  [unwired: 2 out]
      }
      n248 = node-c288(w361) -> ()  [unwired: 1 out]
    }
    frame Enabled {
    }
  }
  n249 = node-c288(3 ("Processor")) -> (w118:T22)  [unwired: 3 out]
  n250 = timed-loop "Oscillate Trap/AOM (fishing, debugging)" {
    tunnel: w32 -> [w458]
    tunnel: [w457] -> w123
    timing: w118 -> [_]
    timing-out: [_] -> w117
    stop <- w457 stop-if-true
    n251 = node-c288() -> ()  [unwired: 2 out]
    n252 = event shown="[0] \"Oscillate Set 1\", \"Fish\": Value Change" {
      selector: _ -> [_ _ _]
      dyn-events: _ -> [_ _ _]
      timeout: _ -> [_ _ _]
      tunnel: w458 -> [w465 _ _]
      tunnel: [FALSE ("Stop All") _ w1150] -> w457
      event "Oscillate Set 1", "Fish": Value Change {
        n253 = event-data() -> ()  [unwired: 6 out]
        n254 = local read "Oscillate Set 1"() -> (w464:bool)
        n255 = Or(x=w464, y="Fish") -> (x .or. y?=w462:bool)
        n256 = case shown="True" w462 {
          tunnel: w465 -> [_ w468]
          tunnel: "Fish" -> [_ w466]
          frame False {
          }
          frame True {
            n257 = case shown="True" w466 {
              selector: w466 -> [w471 w472]
              tunnel: [w471 w472] -> w467
              frame False {
              }
              frame True {
                w473 = FALSE ("Tether")
                n258 = local write "Scan axis 2"(TRUE) -> ()
                n259 = local write "Tether"(w473) -> ()
                n260 = local write "Hysteresis"(w473) -> ()
                n261 = local write "Multiple tether"(w473) -> ()
                n262 = local write "Bad fit"(w473) -> ()
                n263 = local write "Good tether"(w473) -> ()
                n264 = property on="Trap D (MHz)" class="DigNum (strict)"("Val(Sgnl)"="Furthest D (MHz)") -> ()  [unwired: 2 in, 2 out]
                n265 = local read "Flow ON\nduring cal?"() -> (w474:bool)
                n266 = Or(x="Flow ON during \nfishing?", y=w474) -> (x .or. y?=w475:bool)
                n267 = Wait (ms)(milliseconds to wait=u32 500) -> ()  [unwired: 1 out]
                n268 = property on="Sample Channel\nFlow" class="Bool (strict)"("Val(Sgnl)"=w475) -> ()  [unwired: 2 in, 2 out]
              }
            }
            n269 = node-c288() -> (w470:T22)  [unwired: 4 out]
            n270 = timed-loop "Oscillate AOD" {
              timing: w470 -> [_]
              timing-out: [_] -> w469
              tunnel: w468 -> [w487]
              tunnel: w467 -> [w481]
              i -> [w489]
              stop <- w480 stop-if-true
              n271 = node-c288() -> (w488:i64)  [unwired: 1 out]
              n272 = flat-sequence {
                tunnel: w489 -> [w516]
                tunnel: w488 -> [w515]
                tunnel: w487 -> [w494]
                tunnel: w481 -> [w497]
                tunnel: [w497] -> w486
                tunnel: [w496] -> w485
                tunnel: [w493] -> w484
                tunnel: [w490] -> w482
                tunnel: w486 -> [w559]
                tunnel: w485 -> [w557]
                tunnel: w484 -> [w556]
                tunnel: [w555] -> w483
                tunnel: w482 -> [w554]
                tunnel: [w715] -> w480
                tunnel: w483 -> [w714]
                frame #0 {
                  n273 = Divide(x=w515, y=i64 1000) -> (x/y=w510:dbl)
                  n274 = Multiply(x=w510, y=w516) -> (x*y=w512:dbl)
                  n275 = local read "BD 1 Frequency 2 (MHz)"() -> (w495:dbl)
                  n276 = Multiply(x="Osc. freq. (Hz)", y=6.283185307179586) -> (x*y=w513:dbl)
                  n277 = Multiply(x=w513, y=w512) -> (x*y=w492:dbl)
                  n278 = local read "BD 1 Frequency 1 (MHz)"() -> (w500:dbl)
                  n279 = local read "BD 2 Frequency 1 (MHz)"() -> (w499:dbl)
                  n280 = case shown="True" w497 {
                    tunnel: w492 -> [w522 w527]
                    tunnel: w500 -> [_ w538]
                    tunnel: w495 -> [_ w539]
                    tunnel: [w519 w533] -> w498
                    tunnel: [FALSE w530] -> w493
                    tunnel: [0.0 w523] -> w490
                    frame False {
                      n281 = Sine(x=w522) -> (sin(x)=w520:dbl)
                      n282 = Multiply(x=w520, y="Osc. amp. (MHz)") -> (x*y=w519:dbl)
                    }
                    frame True {
                      n283 = Cosine(x=w527) -> (cos(x)=w542:dbl)
                      n284 = Subtract(x=w539, y=w538) -> (x-y=w537:dbl)
                      n285 = Decrement(x=w542) -> (x-1=w541:dbl)
                      n286 = Subtract(x=w537, y="Closest D (MHz)") -> (x-y=w534:dbl)
                      n287 = Divide(x=w541, y=-2.0) -> (x/y=w535:dbl)
                      n288 = Multiply(x=w535, y=w534) -> (x*y=w533:dbl)
                      n289 = local read "Vec Mean of T1 T2"() -> (w529:dbl[])
                      n290 = Greater?(x=w529, y="Stop F (pN)") -> (0:w531:bool[])
                      n291 = Or Array Elements(Boolean array=w531) -> (logical OR=w530:bool)
                      n292 = Divide(x=w527, y=6.283185307179586) -> (x/y=w526:dbl)
                      n293 = Round Toward +Infinity(x=w526) -> (ceil(x): smallest int >= x=w523:dbl)
                      "Attempts" <- w523
                      n294 = Greater?(x=w523, y="Attempt Limit") -> (0:w525:bool)
                      n295 = case shown="True" w525 {
                        frame False {
                        }
                        frame True {
                          n296 = local write "Fish"(FALSE ("Fish for Tether")) -> ()
                          n297 = local read "Messages"() -> (w544:string)
                          n298 = flat-sequence {
                            frame #0 {
                              n299 = call <vilib>:"Beep.vi"("use system alert? (T)"=FALSE, "duration (msec)"=u32 200, "frequency (Hz)"=u32 500) -> ()  [unwired: 9 out]
                            }
                            frame #1 {
                              n300 = Wait (ms)(milliseconds to wait=u32 100) -> ()  [unwired: 1 out]
                            }
                            frame #2 {
                              n301 = call <vilib>:"Beep.vi"("use system alert? (T)"=FALSE, "duration (msec)"=u32 200, "frequency (Hz)"=u32 500) -> ()  [unwired: 9 in]
                            }
                          }
                          n302 = call "Update messages.vi"("Message to add"="Tether fishing timeout." ("Messages"), "Old message string"=w544) -> ("New message string"=→"Messages":string)
                        }
                      }
                    }
                  }
                  n303 = Select(t=w500, s="Scan axis 2", f=w499) -> (s? t:f=w503:dbl)
                  n304 = Add(x=w498, y=w503) -> (x+y=w496:dbl)
                  n305 = Select(t=w496, s="Scan axis 2", f=w500) -> (s? t:f=w506:dbl)
                  n306 = Select(t=w499, s="Scan axis 2", f=w496) -> (s? t:f=w505:dbl)
